vi "Read Map DVR.vi"(8 "error in (no error)":errorcluster, 11 "Permanent Wall in":refnum<class "Permanent Wall.lvclass">) -> (0 "error out":errorcluster, 2 "Map DVR":T1, 3 "Permanent Wall out":refnum<class "Permanent Wall.lvclass">)   [LabVIEW 2015, in "Permanent Wall.lvclass"]
uses:
  Permanent Wall.lvclass
  Common/Map DVR.ctl
  Common/Location Data.ctl
  Permanent Wall.lvclass/Permanent Wall.ctl
  Common/Common.lvlib
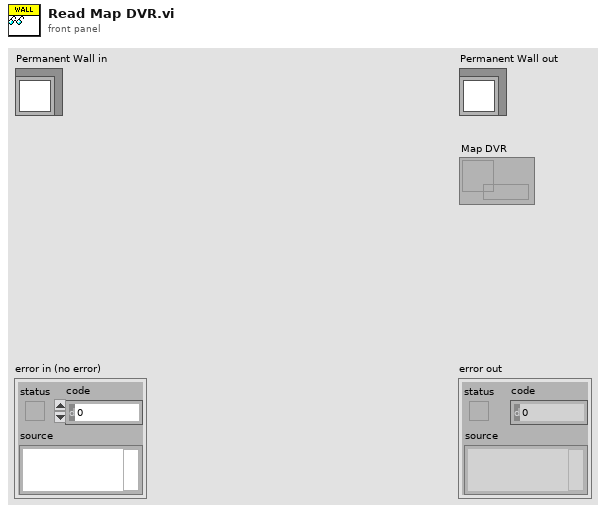
[diagram p1: front panel]
types:
  T1 = typedef "Common.lvlib/Map DVR.ctl" = refnum<data-value>
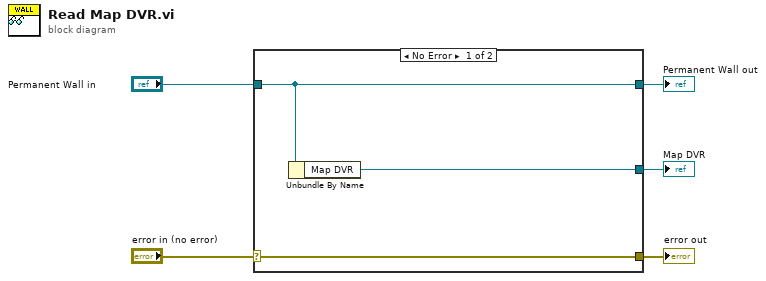
[diagram p0: block diagram]
diagram:
  n1 = case shown="No Error" "error in (no error)" {
    selector: "error in (no error)" -> [w8 w9]
    tunnel: [w8 w9] -> w4
    tunnel: [w7 w10] -> w2
    tunnel: "Permanent Wall in" -> [w7 w10]
    tunnel: [w6 _] -> w1
    frame No Error {
      n2 = Unbundle By Name(w7) -> ("Map DVR"=w6:T1)
    }
    frame Error {
    }
  }
  "error out" <- w4
  "Permanent Wall out" <- w2
  "Map DVR" <- w1
